vi "shift standard cluster.vi"(7 "read write shift":string(combo), 8 "error in":errorcluster, 10 "cycle results cluster In":T1) -> (0 "error out":errorcluster, 2 "cycle results cluster out":T1)   [LabVIEW 2016]
doc: "Shift register used to transport data from one analysis vi to another"
uses:
  controls/cycle results control.ctl
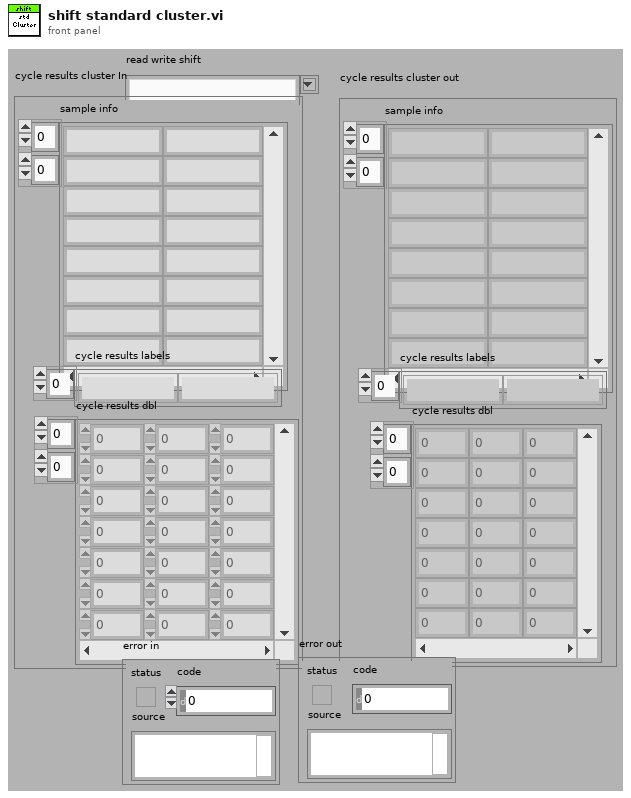
[diagram p1: front panel]
types:
  T1 = typedef "cycle results control.ctl" = cluster{"sample info":string[][], "cycle results labels":string[], "cycle results dbl":dbl[][]}
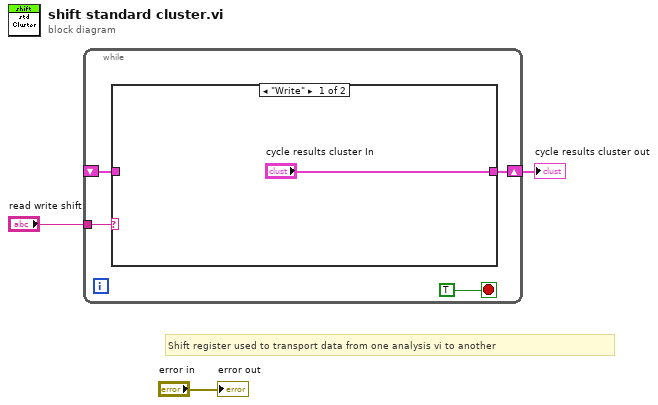
[diagram p0: block diagram]
diagram:
  # "Shift register used to transport data from one analysis vi to another"
  n1 = while {
    tunnel: "read write shift" -> [w7]
    shift-right: [w6] -> w2
    shift-left: _ -> [w4]
    stop <- TRUE stop-if-true
    n2 = case shown="\"Write\"" w7 {
      tunnel: ["cycle results cluster In" w9] -> w6
      tunnel: w4 -> [_ w9]
      frame "Write" {
      }
      frame "Read", Default {
      }
    }
  }
  "cycle results cluster out" <- w2
  "error out" <- "error in"
